vi "arrays.vi"() -> ()   [LabVIEW 2020]
uses:
  8cb993e0-1817-489b-9034-5cf87d91466b.vi
  9d1ead81-767c-4c11-aa30-6a7ff094f613.vi
panel:
  out "array out 2":dbl[](array[numeric])
  out "array out":dbl[](array[numeric])
  out "index of element":i32
  out "min index(es)":i32
  out "min value":dbl
  out "max index(es)":i32
  out "max value":dbl
  out "appended array":dbl[](array[numeric])
  in  "Numeric 4":dbl
  in  "Numeric 3":dbl
  in  "Numeric 2":dbl
  in  "Numeric":dbl
  out "initialized array 3":string[](array[string])
  out "initialized array 2":bool[](array[boolean])
  out "initialized array":i32[](array[numeric])
  out "subarray":u16[](array[numeric])
  out "output array 2":u16[](array[numeric])
  in  "Tank":u8(slide) scale=0.0..10.0
  in  "Meter":u8(knob) scale=0.0..10.0
  in  "Array 4":u16[](array[numeric])
  out "element 5":string
  in  "Array 3":string[](array[string])
  out "output array":bool[](array[boolean])
  in  "Array 2":bool[](array[boolean])
  out "size(s)":i32
  out "element 4":dbl
  out "element 3":dbl
  out "element 2":dbl
  out "element":dbl
  in  "Array":dbl[](array[slide]) scale=0.0..10.0
  # "Arrays"
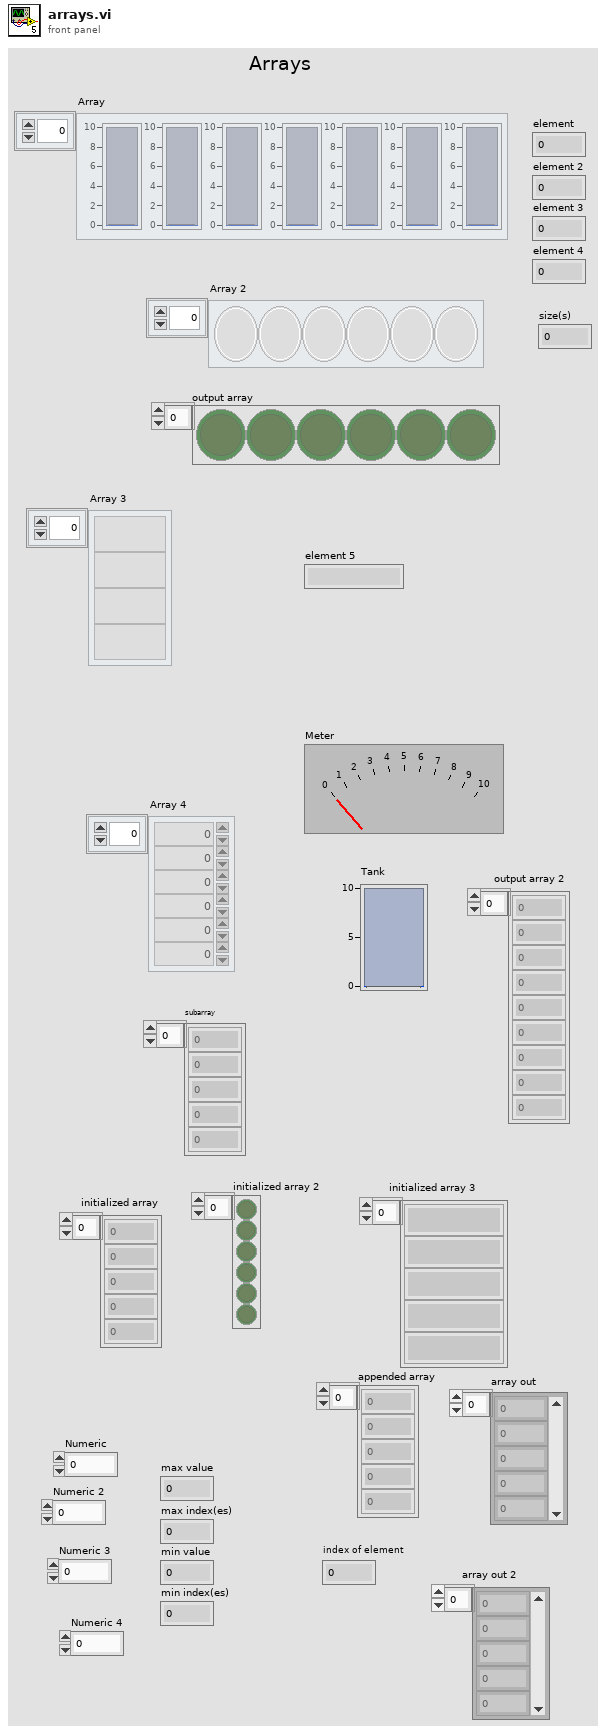
[diagram p1: front panel]
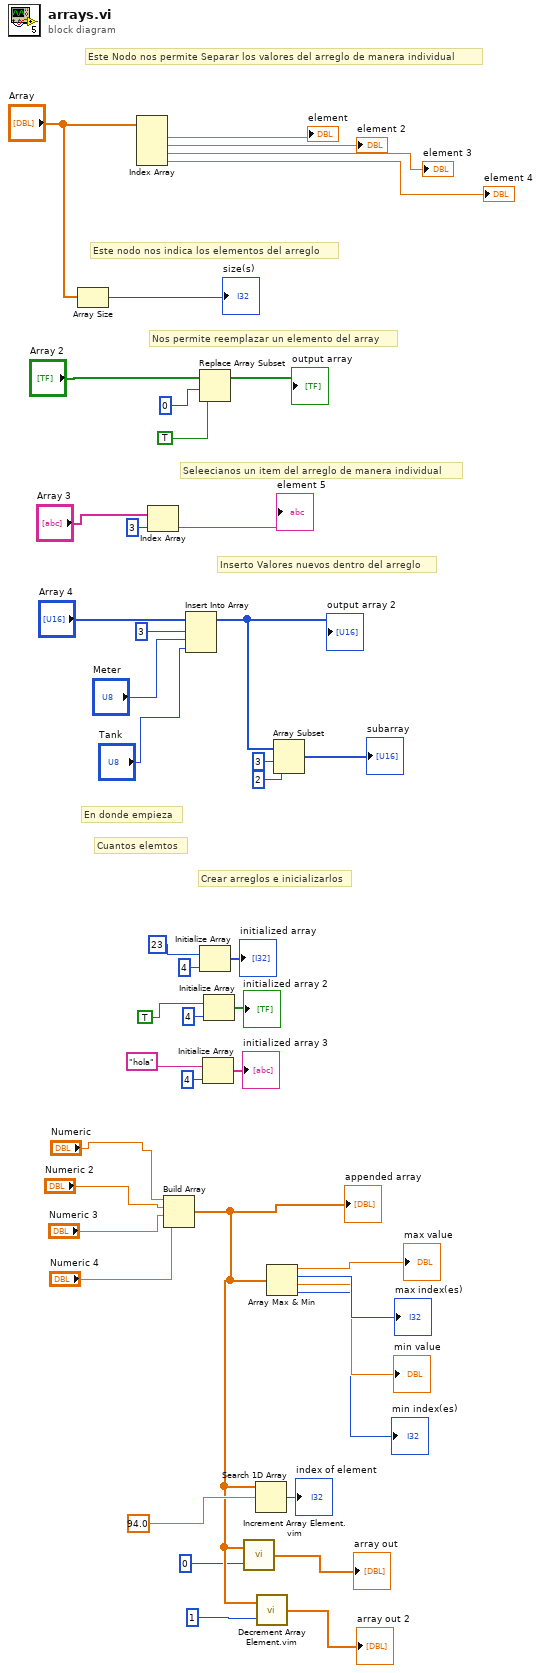
[diagram p0: block diagram]
diagram:
  # "Crear arreglos e inicializarlos"
  # "Cuantos elemtos"
  # "En donde empieza"
  # "Inserto Valores nuevos dentro del arreglo"
  # "Seleecianos un item del arreglo de manera individual"
  # "Nos permite reemplazar un elemento del array"
  # "Este nodo nos indica los elementos del arreglo"
  # "Este Nodo nos permite Separar los valores del arreglo de manera individual"
  n1 = Array Size(array="Array") -> (size(s)=→"size(s)":i32)
  n2 = Index Array(array="Array") -> (element #1=→"element":dbl, element #2=→"element 2":dbl, element #3=→"element 3":dbl, element #4=→"element 4":dbl)  [unwired: 4 in]
  n3 = Index Array(array="Array 3", index=3) -> (element=→"element 5":string)
  n4 = Build Array("Numeric", "Numeric 2", "Numeric 3", "Numeric 4") -> (w5:dbl[])
  "appended array" <- w5
  n5 = Insert Into Array(array="Array 4", index=3, new element #1="Meter", new element #2="Tank") -> (w28:u16[])
  "output array 2" <- w28
  n6 = Replace Array Subset(array="Array 2", new element=TRUE ("new element/subarray"), index=0) -> (→"output array":bool[])
  n7 = Initialize Array(23, 4 ("dimension size")) -> (→"initialized array":i32[])
  n8 = Initialize Array("hola", 4 ("dimension size")) -> (→"initialized array 3":string[])
  n9 = Initialize Array(TRUE, 4 ("dimension size")) -> (→"initialized array 2":bool[])
  n10 = call "Increment Array Element.vim"("index"=0, "array in"=w5) -> ("array out"=→"array out":dbl[])
  n11 = Search 1D Array(1D array=w5, element=94.0) -> (index of element=→"index of element":i32)  [unwired: 1 in]
  n12 = call "Decrement Array Element.vim"("index"=1, "array in"=w5) -> ("array out"=→"array out 2":dbl[])
  n13 = Array Max & Min(array=w5) -> (max value=→"max value":dbl, max index (indices)=→"max index(es)":i32, min value=→"min value":dbl, min index (indices)=→"min index(es)":i32)
  n14 = Array Subset(array=w28, index=3, length=2) -> (→"subarray":u16[])
